vi "Get Polymorphic.vi"   [LabVIEW 2020, in "NI_VIAnCFGDataStructure.lvlib" / "Tree.lvclass"]
doc: "Polymorphic instance of the Get method. Select the appropraite instance to work with or allow this method to adapt automatically."
uses:
  <vilib>/addons/analyzer/VIAnCFGDataStructure/Tree Manager/Tree.lvclass
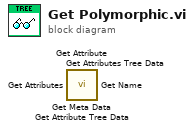
[diagram p0: block diagram]
diagram:
  n1 = call <vilib>:"Get Meta Data.vi"() -> ()  [unwired: 9 in, 3 out]
  n2 = call <vilib>:"Get Attributes Tree Data.vi"() -> ()  [unwired: 8 in, 4 out]
  n3 = call <vilib>:"Get Attributes.vi"() -> ()  [unwired: 8 in, 4 out]
  n4 = call <vilib>:"Get Name.vi"() -> ()  [unwired: 9 in, 3 out]
  n5 = call <vilib>:"Get Attribute Tree Data.vi"() -> ()  [unwired: 8 in, 4 out]
  n6 = call <vilib>:"Get Attribute.vi"() -> ()  [unwired: 8 in, 4 out]
